vi "MiniCTA.vi"() -> ()   [LabVIEW 2020]
uses:
  controls/DIPSingleRadioButton.ctl
  controls/DIPBankRadioButton.ctl
  <vilib>/Utility/NIReport.llb/NI_ReportGenerationCore.lvlib
  <vilib>/printing/EasyPrintingControls.llb/report_type.ctl
  <vilib>/printing/EasyPrintingControls.llb/orientation.ctl
  <vilib>/printing/EasyPrintingControls.llb/panel_scaling_for_page.ctl
  <vilib>/printing/EasyPrintingControls.llb/margin_values.ctl
  <vilib>/printing/EasyPrintingControls.llb/measurement_system.ctl
  <vilib>/printing/EasyPrintingControls.llb/margins.ctl
  <vilib>/printing/EasyPrintingControls.llb/printing_method.ctl
  <vilib>/printing/EasyPrintingControls.llb/color_or_monochrome.ctl
  <vilib>/printing/EasyPrintingControls.llb/printer_options.ctl
  <vilib>/printing/EasyPrintingControls.llb/page_headers.ctl
  <vilib>/printing/EasyPrintingControls.llb/page_header_content_options.ctl
  <vilib>/printing/EasyPrintingControls.llb/page_header_options.ctl
  <vilib>/printing/EasyPrintingControls.llb/layout_options.ctl
  <vilib>/printing/EasyPrintingControls.llb/list_which_controls.ctl
  <vilib>/printing/EasyPrintingControls.llb/custom_contents_options.ctl
  <vilib>/printing/EasyPrinting.llb/Easy Print VI Panel or Documentation (path).vi
panel:
  in  "Tab Control":T1(tab)
  in  "Cable Length (m)":dbl=4.0 min=4.0 max=20.0 step=1.0
  out "SW1":T2
  out "SW2":T2
  out "SW3":T2
  out "ShortOK":bool
  out "ProbeOK":bool
  in  "Shorted Resistance":dbl min=0.0 max=2.0 step=0.1 format="%.2g"
  in  "Total Resistance":dbl min=0.0 max=100.0 step=0.1 format="%.2g"
  out "AllOK?":bool
  out "Cable Resistance":dbl format="%.2g"
  out "Filament\nHot Resistance":dbl format="%.2g"
  in  "Overheat":dbl=1.5
  out "Filament\nCold Resistance":dbl format="%.2g"
  out "TargetTotal\nHotResistance":dbl
  out "BridgeSetting":dbl
  out "Rbin":dbl
  out "SW1remainder":dbl
  out "n160":i32
  out "n20":i32
  out "SW2remainder":dbl
  out "n1.4":i32
  out "SW3remainder":dbl
  in  "alpha":dbl=0.0039
  out "Failed recipients":string[](array[string])
  in  "print?":bool
  in  "Recipients":string[](array[string])=["ttech@cppwind.com"]
  in  "Stop Button":bool
  in  "email?":bool
  # "1. Connect probe holder (sting or pigtail type) to 4-10m or 10-20m probe cable; SET DIP  SW1- 3 OR 4 appropriately\n2. Insert shorting probe.\n2. Use CEM DT-5302 (or alternative) Low Resistance Tester on 40 Ohm range to measure shorted holder and cable resistance, and enter displayed value on \"Basic\" tab.\n3. Remove shorting probe and insert hotfilm probe.\n4. Measure total resistance and enter displayed value on \"Basic\" tab, again using the 40 Ohm range setting. CAUTION! The 4 and 400 milliohm settings on the CEM DT-5302 drive large enough currents to damage the probe after a few seconds by heat dissipated through the probe.\n5. Set DIP switches as shown - a  dot indicating the switch should be pushed on that side.\n6. Connect the probe cable to the anemometer's \"Probe\" connection.\n7. Power up the bridge by plugging in PSU.\n\nOnly connect probe AFTER switches are set correctly. Power down before unplugging probe."
  # "="
  # "+"
  # "="
  # "X"
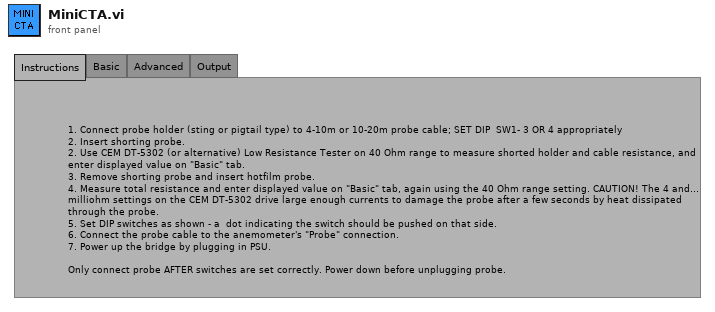
[diagram p1: front panel]
types:
  T1 = enum32{"Instructions", "Basic", "Advanced", "Output"}
  T2 = typedef "DIPBankRadioButton.ctl" = T3[]
  T3 = typedef "DIPSingleRadioButton.ctl" = enum32{"Radio Selection 1", "Radio Selection 2"}
  T4 = typedef "NI_ReportGenerationCore.lvlib/custom_contents_options.ctl" = cluster{"include VI connector and icon":bool, "include VI description":bool, "include front panel":bool, "surround front panel with border":bool, "list of controls options":cluster{"include list of controls":bool, "list which controls?":T5, "include control descriptions?":bool, "include control data types?":bool}, "block diagram options":cluster{"include block diagram":bool, "hidden frames":bool, "ordered (repeat from higher level if nested)":bool}, "include VI hierarchy":bool, "include list of subVIs":bool, "include VI history":bool, "include Express VI configuration information":bool}
  T5 = typedef "NI_ReportGenerationCore.lvlib/list_which_controls.ctl" = u16
  T6 = typedef "NI_ReportGenerationCore.lvlib/layout_options.ctl" = cluster{"orientation (unchanged)":T7, "panel scaling for page (unchanged)":T8, "margins":T9, "printer options":T12, "page header options":T15}
  T7 = typedef "NI_ReportGenerationCore.lvlib/orientation.ctl" = u16
  T8 = typedef "NI_ReportGenerationCore.lvlib/panel_scaling_for_page.ctl" = u16
  T9 = typedef "NI_ReportGenerationCore.lvlib/margins.ctl" = cluster{"override VI margins (false)":bool, "margins (1.00)":T10, "measurement system (default)":T11}
  T10 = typedef "NI_ReportGenerationCore.lvlib/margin_values.ctl" = cluster{"top":dbl, "left":dbl, "right":dbl, "bottom":dbl}
  T11 = typedef "NI_ReportGenerationCore.lvlib/measurement_system.ctl" = u16
  T12 = typedef "NI_ReportGenerationCore.lvlib/printer_options.ctl" = cluster{"destination printer name (current)":string, "printing method (unchanged)":T13, "color or monochrome (unchanged)":T14}
  T13 = typedef "NI_ReportGenerationCore.lvlib/printing_method.ctl" = u16
  T14 = typedef "NI_ReportGenerationCore.lvlib/color_or_monochrome.ctl" = u16
  T15 = typedef "NI_ReportGenerationCore.lvlib/page_header_options.ctl" = cluster{"page headers (unchanged)":T16, "page header content options":T17}
  T16 = typedef "NI_ReportGenerationCore.lvlib/page_headers.ctl" = u16
  T17 = typedef "NI_ReportGenerationCore.lvlib/page_header_content_options.ctl" = cluster{"Include VI Name":bool, "Include VI Path":bool, "Include Last Modification Date":bool, "Include Date Printed":bool, "Include Page Number":bool, "Include VI Icon":bool}
  T18 = typedef "NI_ReportGenerationCore.lvlib/report_type.ctl" = u16
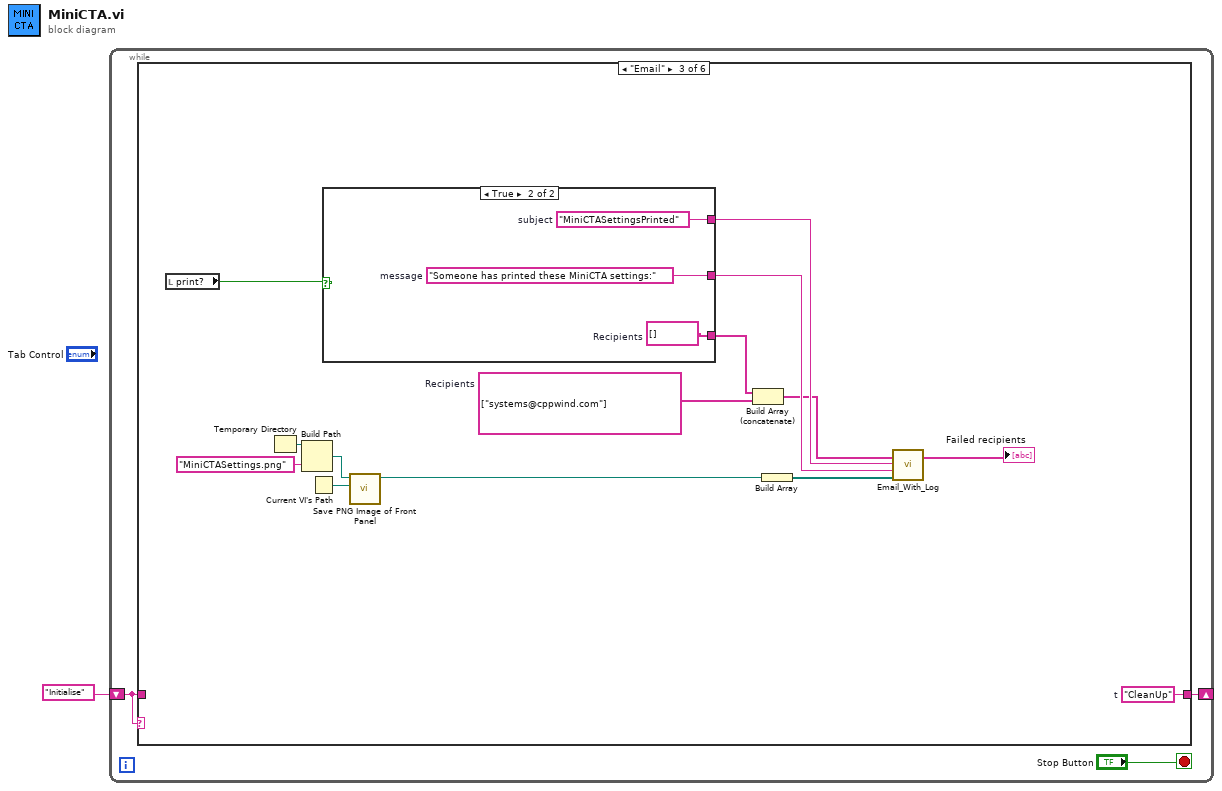
[diagram p0: block diagram]
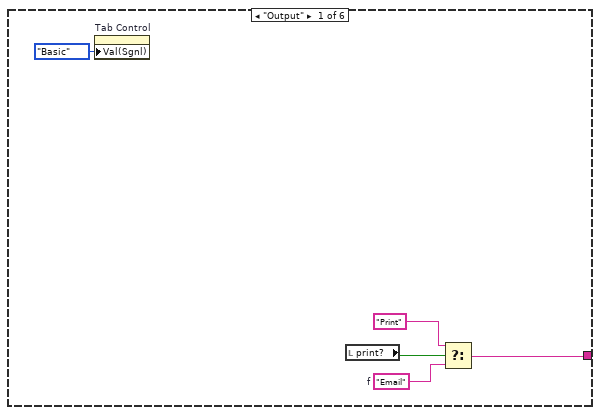
[diagram p2: hidden frame]
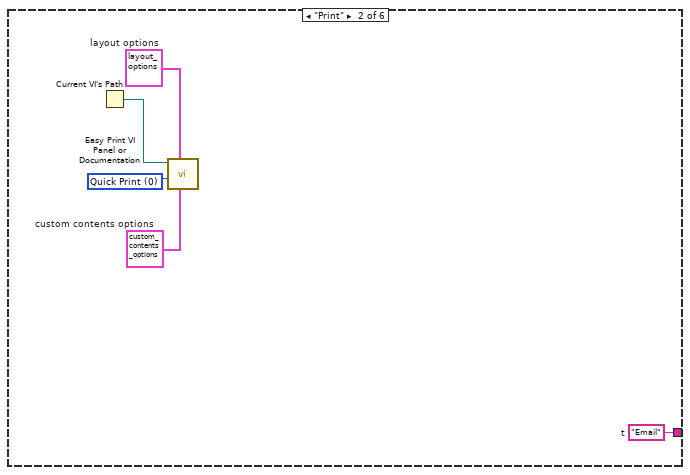
[diagram p3: hidden frame]
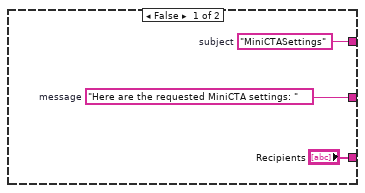
[diagram p4: hidden frame]
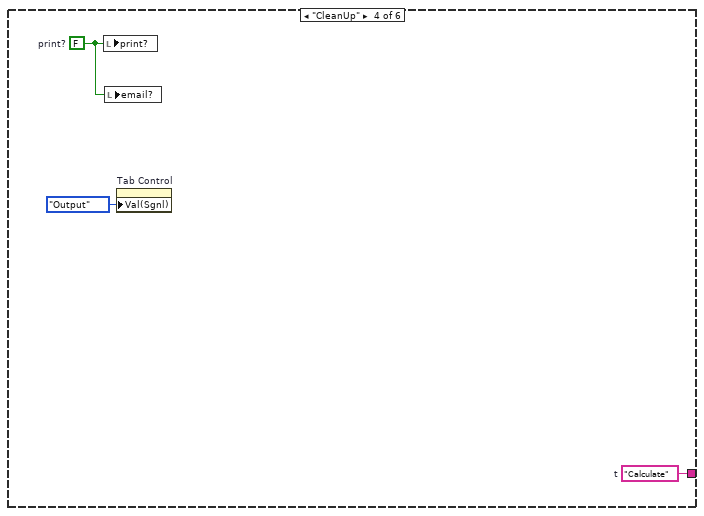
[diagram p5: hidden frame]
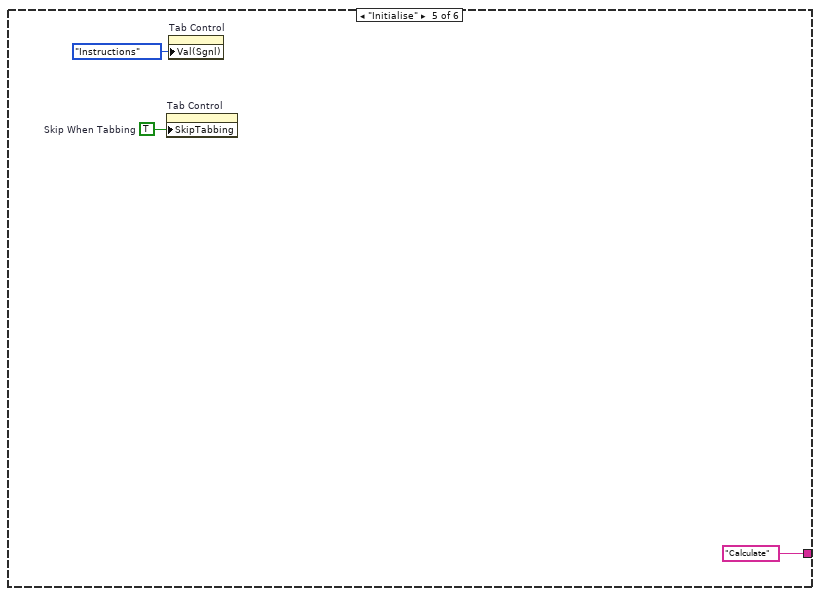
[diagram p6: hidden frame]
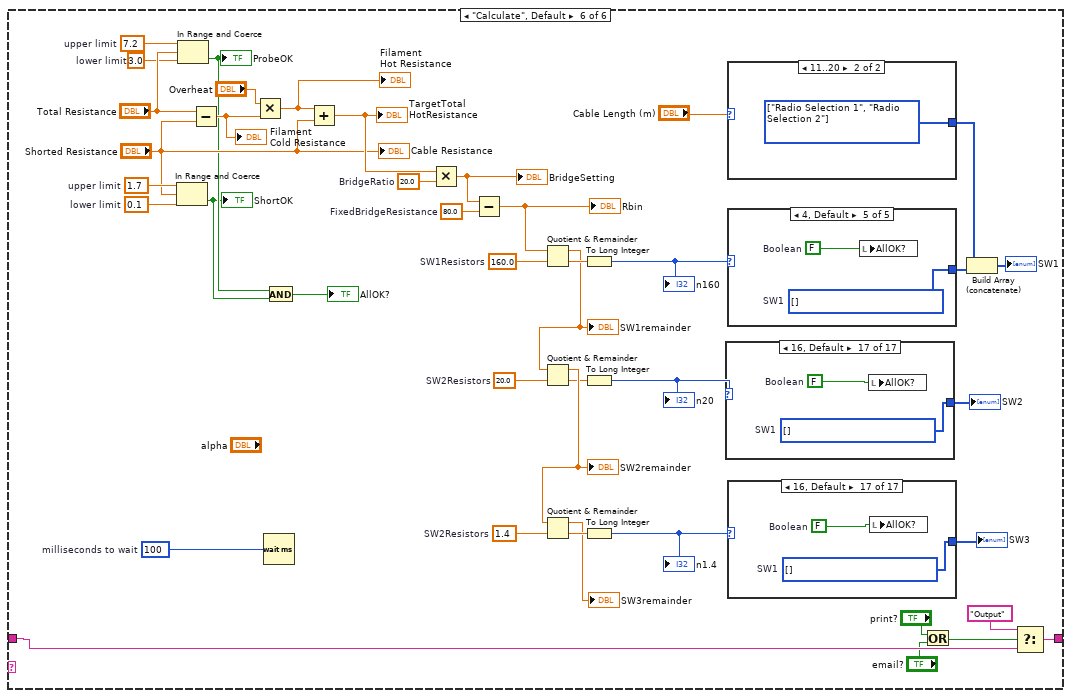
[diagram p7: hidden frame]
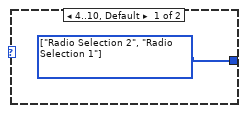
[diagram p8: hidden frame]
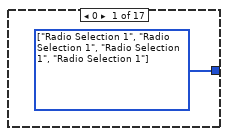
[diagram p9: hidden frame]
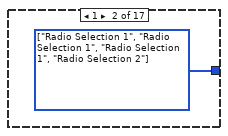
[diagram p10: hidden frame]
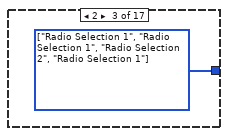
[diagram p11: hidden frame]
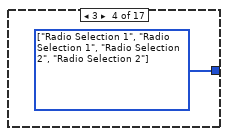
[diagram p12: hidden frame]
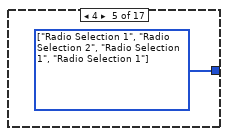
[diagram p13: hidden frame]
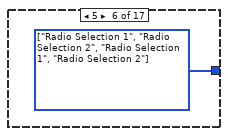
[diagram p14: hidden frame]
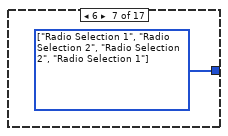
[diagram p15: hidden frame]
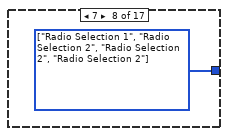
[diagram p16: hidden frame]
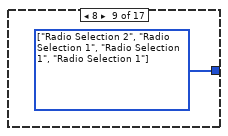
[diagram p17: hidden frame]
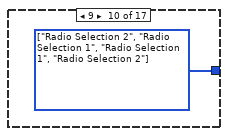
[diagram p18: hidden frame]
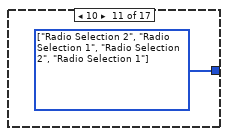
[diagram p19: hidden frame]
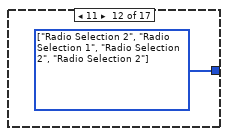
[diagram p20: hidden frame]
diagram:
  n1 = while {
    shift-right: [w2] -> _
    shift-left: "Initialise" -> [w3]
    stop <- "Stop Button" stop-if-true
    n2 = case shown="\"Email\"" w3 {
      tunnel: w3 -> [_ _ _ _ _ w50]
      tunnel: [w8 w13 w28 w36 "Calculate" w51] -> w2
      frame "Output" {
        w5 = "Email"  # f
        n3 = property on="Tab Control" class="TabCtl (strict)"("Val(Sgnl)"=T1."Basic" ("Value (Signaling)")) -> ()  [unwired: 2 in, 2 out]
        n4 = local read "print?"() -> (w7:bool)
        n5 = Select(t="Print", s=w7, f=w5) -> (s? t:f=w8:string)
      }
      frame "Print" {
        w10 = T4 {"include VI connector and icon"=FALSE, "include VI description"=FALSE, "include front panel"=FALSE, "surround front panel with border"=FALSE, "list of controls options"={"include list of controls"=FALSE, "list which controls?"=0, "include control descriptions?"=FALSE, "include control data types?"=FALSE}, "block diagram options"={"include block diagram"=FALSE, "hidden frames"=FALSE, "ordered (repeat from higher level if nested)"=FALSE}, "include VI hierarchy"=FALSE, "include list of subVIs"=FALSE, "include VI history"=FALSE, "include Express VI configuration information"=FALSE}  # custom contents options
        w11 = T6 {"orientation (unchanged)"=0, "panel scaling for page (unchanged)"=0, "margins"={"override VI margins (false)"=FALSE, "margins (1.00)"={"top"=1.0, "left"=1.0, "right"=1.0, "bottom"=1.0}, "measurement system (default)"=0}, "printer options"={"destination printer name (current)"="", "printing method (unchanged)"=0, "color or monochrome (unchanged)"=0}, "page header options"={"page headers (unchanged)"=1, "page header content options"={"Include VI Name"=FALSE, "Include VI Path"=FALSE, "Include Last Modification Date"=FALSE, "Include Date Printed"=TRUE, "Include Page Number"=FALSE, "Include VI Icon"=FALSE}}}  # layout options
        w12 = T18 0 items=["Quick Print", "Standard Report", "HTML", "Word", "Excel"] ("report type (Quick Print)")
        w13 = "Email"  # t
        n6 = Current VI's Path() -> (path=w14:path)
        n7 = call-poly <vilib>:"Easy Print VI Panel or Documentation.vi"("custom contents options"=w10, "layout options"=w11, "report type (Quick Print)"=w12, "VI path"=w14) -> ()  [unwired: 6 in, 2 out]
      }
      frame "Email" {
        w24 = string[] ["systems@cppwind.com"]  # Recipients
        w28 = "CleanUp"  # t
        n8 = local read "print?"() -> (w21:bool)
        n9 = Temporary Directory() -> (w27:path)
        n10 = Build Path(base path=w27, name or relative path="MiniCTASettings.png") -> (appended path=w26:path)
        n11 = Current VI's Path() -> (path=w22:path)
        n12 = case shown="True" w21 {
          tunnel: ["Recipients" w34] -> w23
          tunnel: [w30 w33] -> w18
          tunnel: [w29 w32] -> w19
          frame False {
            w29 = "Here are the requested MiniCTA settings: "  # message
            w30 = "MiniCTASettings"  # subject
          }
          frame True {
            w32 = "Someone has printed these MiniCTA settings:"  # message
            w33 = "MiniCTASettingsPrinted"  # subject
            w34 = string[] []  # Recipients
          }
        }
        n13 = call "Save PNG Image of Front Panel.vi"("VI Path"=w22, "File Path In"=w26) -> ("File Path Out"=w15:path)  [unwired: 8 in, 1 out]
        n14 = Build Array (concatenate)(w23, w24) -> (w17:string[])
        n15 = Build Array(w15) -> (w20:path[])
        n16 = call "Email_With_Log.vi"("recipients"=w17, "subject ([No Subject])"=w18, "message"=w19, "attachments"=w20) -> ("invalid recipients"=→"Failed recipients":string[])  [unwired: 1 in, 1 out]
      }
      frame "CleanUp" {
        w36 = "Calculate"  # t
        w37 = FALSE  # print?
        n17 = local write "print?"(w37) -> ()
        n18 = local write "email?"(w37) -> ()
        n19 = property on="Tab Control" class="TabCtl (strict)"("Val(Sgnl)"=T1."Output" ("Value (Signaling)")) -> ()  [unwired: 2 in, 2 out]
      }
      frame "Initialise" {
        w38 = TRUE  # Skip When Tabbing
        n20 = property on="Tab Control" class="TabCtl (strict)"("SkipTabbing"=w38) -> ()  [unwired: 2 in, 2 out]
        n21 = property on="Tab Control" class="TabCtl (strict)"("Val(Sgnl)"=T1."Instructions" ("Value (Signaling)")) -> ()  [unwired: 2 in, 2 out]
      }
      frame "Calculate", Default {
        w55 = 7.2  # upper limit
        w56 = 3.0  # lower limit
        w58 = 0.1  # lower limit
        w59 = 1.7  # upper limit
        w60 = u32 100  # milliseconds to wait
        w69 = 1.4  # SW2Resistors
        w72 = 20.0  # SW2Resistors
        w75 = 160.0  # SW1Resistors
        w77 = 80.0  # FixedBridgeResistance
        w79 = 20.0  # BridgeRatio
        n22 = In Range and Coerce(upper limit=w59, x="Shorted Resistance", lower limit=w58) -> (In Range?=w42:bool)  [unwired: 1 out]
        "ShortOK" <- w42
        n23 = In Range and Coerce(upper limit=w55, x="Total Resistance", lower limit=w56) -> (In Range?=w43:bool)  [unwired: 1 out]
        "ProbeOK" <- w43
        n24 = Subtract(x="Total Resistance", y="Shorted Resistance") -> (x-y=w82:dbl)
        "Filament\nCold Resistance" <- w82
        n25 = Multiply(x="Overheat", y=w82) -> (x*y=w45:dbl)
        "Filament\nHot Resistance" <- w45
        n26 = Wait (ms)(milliseconds to wait=w60) -> ()  [unwired: 1 out]
        n27 = And(x=w43, y=w42) -> (x .and. y?=→"AllOK?":bool)
        n28 = Add(x=w45, y="Shorted Resistance") -> (x+y=w80:dbl)
        "TargetTotal\nHotResistance" <- w80
        n29 = Multiply(x=w80, y=w79) -> (x*y=w78:dbl)
        "BridgeSetting" <- w78
        n30 = Subtract(x=w78, y=w77) -> (x-y=w76:dbl)
        "Rbin" <- w76
        n31 = Quotient & Remainder(x=w76, y=w75) -> (x-y*floor(x/y)=w71:dbl, floor(x/y)=w74:dbl)
        "SW1remainder" <- w71
        n32 = Quotient & Remainder(x=w71, y=w72) -> (x-y*floor(x/y)=w68:dbl, floor(x/y)=w65:dbl)
        "SW2remainder" <- w68
        n33 = Quotient & Remainder(x=w68, y=w69) -> (x-y*floor(x/y)=→"SW3remainder":dbl, floor(x/y)=w63:dbl)
        n34 = To Long Integer(number=w74) -> (32bit integer=w66:i32)
        "n160" <- w66
        n35 = To Long Integer(number=w65) -> (32bit integer=w64:i32)
        "n20" <- w64
        n36 = To Long Integer(number=w63) -> (32bit integer=w62:i32)
        "n1.4" <- w62
        n37 = case shown="16, Default" w64 {
          tunnel: [w103 w104 w105 w106 w107 w108 w109 w110 w111 w112 w113 w114 w115 w116 w117 w118 w120] -> w70
          frame 0 {
            w103 = T2 [enum."Radio Selection 1", enum."Radio Selection 1", enum."Radio Selection 1", enum."Radio Selection 1"] items=["Radio Selection 1", "Radio Selection 2"] ("SW1")
          }
          frame 1 {
            w104 = T2 [enum."Radio Selection 1", enum."Radio Selection 1", enum."Radio Selection 1", enum."Radio Selection 2"] items=["Radio Selection 1", "Radio Selection 2"] ("SW1")
          }
          frame 2 {
            w105 = T2 [enum."Radio Selection 1", enum."Radio Selection 1", enum."Radio Selection 2", enum."Radio Selection 1"] items=["Radio Selection 1", "Radio Selection 2"] ("SW1")
          }
          frame 3 {
            w106 = T2 [enum."Radio Selection 1", enum."Radio Selection 1", enum."Radio Selection 2", enum."Radio Selection 2"] items=["Radio Selection 1", "Radio Selection 2"] ("SW1")
          }
          frame 4 {
            w107 = T2 [enum."Radio Selection 1", enum."Radio Selection 2", enum."Radio Selection 1", enum."Radio Selection 1"] items=["Radio Selection 1", "Radio Selection 2"] ("SW1")
          }
          frame 5 {
            w108 = T2 [enum."Radio Selection 1", enum."Radio Selection 2", enum."Radio Selection 1", enum."Radio Selection 2"] items=["Radio Selection 1", "Radio Selection 2"] ("SW1")
          }
          frame 6 {
            w109 = T2 [enum."Radio Selection 1", enum."Radio Selection 2", enum."Radio Selection 2", enum."Radio Selection 1"] items=["Radio Selection 1", "Radio Selection 2"] ("SW1")
          }
          frame 7 {
            w110 = T2 [enum."Radio Selection 1", enum."Radio Selection 2", enum."Radio Selection 2", enum."Radio Selection 2"] items=["Radio Selection 1", "Radio Selection 2"] ("SW1")
          }
          frame 8 {
            w111 = T2 [enum."Radio Selection 2", enum."Radio Selection 1", enum."Radio Selection 1", enum."Radio Selection 1"] items=["Radio Selection 1", "Radio Selection 2"] ("SW1")
          }
          frame 9 {
            w112 = T2 [enum."Radio Selection 2", enum."Radio Selection 1", enum."Radio Selection 1", enum."Radio Selection 2"] items=["Radio Selection 1", "Radio Selection 2"] ("SW1")
          }
          frame 10 {
            w113 = T2 [enum."Radio Selection 2", enum."Radio Selection 1", enum."Radio Selection 2", enum."Radio Selection 1"] items=["Radio Selection 1", "Radio Selection 2"] ("SW1")
          }
          frame 11 {
            w114 = T2 [enum."Radio Selection 2", enum."Radio Selection 1", enum."Radio Selection 2", enum."Radio Selection 2"] items=["Radio Selection 1", "Radio Selection 2"] ("SW1")
          }
          frame 12 {
            w115 = T2 [enum."Radio Selection 2", enum."Radio Selection 2", enum."Radio Selection 1", enum."Radio Selection 1"] items=["Radio Selection 1", "Radio Selection 2"] ("SW1")
          }
          frame 13 {
            w116 = T2 [enum."Radio Selection 2", enum."Radio Selection 2", enum."Radio Selection 1", enum."Radio Selection 2"] items=["Radio Selection 1", "Radio Selection 2"] ("SW1")
          }
          frame 14 {
            w117 = T2 [enum."Radio Selection 2", enum."Radio Selection 2", enum."Radio Selection 2", enum."Radio Selection 1"] items=["Radio Selection 1", "Radio Selection 2"] ("SW1")
          }
          frame 15 {
            w118 = T2 [enum."Radio Selection 2", enum."Radio Selection 2", enum."Radio Selection 2", enum."Radio Selection 2"] items=["Radio Selection 1", "Radio Selection 2"] ("SW1")
          }
          frame 16, Default {
            w119 = FALSE  # Boolean
            w120 = T2 [] items=["Radio Selection 1", "Radio Selection 2"]  # SW1
            n38 = local write "AllOK?"(w119) -> ()
          }
        }
        "SW2" <- w70
        n39 = case shown="11..20" "Cable Length (m)" {
          tunnel: [w83 w84] -> w52
          frame 4..10, Default {
            w83 = T2 [enum."Radio Selection 2", enum."Radio Selection 1"] items=["Radio Selection 1", "Radio Selection 2"] ("SW1")
          }
          frame 11..20 {
            w84 = T2 [enum."Radio Selection 1", enum."Radio Selection 2"] items=["Radio Selection 1", "Radio Selection 2"] ("SW1")
          }
        }
        n40 = case shown="4, Default" w66 {
          tunnel: [w121 w122 w123 w124 w126] -> w73
          frame 0 {
            w121 = T2 [enum."Radio Selection 1", enum."Radio Selection 1"] items=["Radio Selection 1", "Radio Selection 2"] ("SW1")
          }
          frame 1 {
            w122 = T2 [enum."Radio Selection 1", enum."Radio Selection 2"] items=["Radio Selection 1", "Radio Selection 2"] ("SW1")
          }
          frame 2 {
            w123 = T2 [enum."Radio Selection 2", enum."Radio Selection 2"] items=["Radio Selection 1", "Radio Selection 2"] ("SW1")
          }
          frame 3 {
            w124 = T2 [enum."Radio Selection 1", enum."Radio Selection 1"] items=["Radio Selection 1", "Radio Selection 2"] ("SW1")
          }
          frame 4, Default {
            w125 = FALSE  # Boolean
            w126 = T2 [] items=["Radio Selection 1", "Radio Selection 2"]  # SW1
            n41 = local write "AllOK?"(w125) -> ()
          }
        }
        n42 = case shown="16, Default" w62 {
          tunnel: [w85 w86 w87 w88 w89 w90 w91 w92 w93 w94 w95 w96 w97 w98 w99 w100 w102] -> w67
          frame 0 {
            w85 = T2 [enum."Radio Selection 1", enum."Radio Selection 1", enum."Radio Selection 1", enum."Radio Selection 1"] items=["Radio Selection 1", "Radio Selection 2"] ("SW1")
          }
          frame 1 {
            w86 = T2 [enum."Radio Selection 1", enum."Radio Selection 1", enum."Radio Selection 1", enum."Radio Selection 2"] items=["Radio Selection 1", "Radio Selection 2"] ("SW1")
          }
          frame 2 {
            w87 = T2 [enum."Radio Selection 1", enum."Radio Selection 1", enum."Radio Selection 2", enum."Radio Selection 1"] items=["Radio Selection 1", "Radio Selection 2"] ("SW1")
          }
          frame 3 {
            w88 = T2 [enum."Radio Selection 1", enum."Radio Selection 1", enum."Radio Selection 2", enum."Radio Selection 2"] items=["Radio Selection 1", "Radio Selection 2"] ("SW1")
          }
          frame 4 {
            w89 = T2 [enum."Radio Selection 1", enum."Radio Selection 2", enum."Radio Selection 1", enum."Radio Selection 1"] items=["Radio Selection 1", "Radio Selection 2"] ("SW1")
          }
          frame 5 {
            w90 = T2 [enum."Radio Selection 1", enum."Radio Selection 2", enum."Radio Selection 1", enum."Radio Selection 2"] items=["Radio Selection 1", "Radio Selection 2"] ("SW1")
          }
          frame 6 {
            w91 = T2 [enum."Radio Selection 1", enum."Radio Selection 2", enum."Radio Selection 2", enum."Radio Selection 1"] items=["Radio Selection 1", "Radio Selection 2"] ("SW1")
          }
          frame 7 {
            w92 = T2 [enum."Radio Selection 1", enum."Radio Selection 2", enum."Radio Selection 2", enum."Radio Selection 2"] items=["Radio Selection 1", "Radio Selection 2"] ("SW1")
          }
          frame 8 {
            w93 = T2 [enum."Radio Selection 2", enum."Radio Selection 1", enum."Radio Selection 1", enum."Radio Selection 1"] items=["Radio Selection 1", "Radio Selection 2"] ("SW1")
          }
          frame 9 {
            w94 = T2 [enum."Radio Selection 2", enum."Radio Selection 1", enum."Radio Selection 1", enum."Radio Selection 2"] items=["Radio Selection 1", "Radio Selection 2"] ("SW1")
          }
          frame 10 {
            w95 = T2 [enum."Radio Selection 2", enum."Radio Selection 1", enum."Radio Selection 2", enum."Radio Selection 1"] items=["Radio Selection 1", "Radio Selection 2"] ("SW1")
          }
          frame 11 {
            w96 = T2 [enum."Radio Selection 2", enum."Radio Selection 1", enum."Radio Selection 2", enum."Radio Selection 2"] items=["Radio Selection 1", "Radio Selection 2"] ("SW1")
          }
          frame 12 {
            w97 = T2 [enum."Radio Selection 2", enum."Radio Selection 2", enum."Radio Selection 1", enum."Radio Selection 1"] items=["Radio Selection 1", "Radio Selection 2"] ("SW1")
          }
          frame 13 {
            w98 = T2 [enum."Radio Selection 2", enum."Radio Selection 2", enum."Radio Selection 1", enum."Radio Selection 2"] items=["Radio Selection 1", "Radio Selection 2"] ("SW1")
          }
          frame 14 {
            w99 = T2 [enum."Radio Selection 2", enum."Radio Selection 2", enum."Radio Selection 2", enum."Radio Selection 1"] items=["Radio Selection 1", "Radio Selection 2"] ("SW1")
          }
          frame 15 {
            w100 = T2 [enum."Radio Selection 2", enum."Radio Selection 2", enum."Radio Selection 2", enum."Radio Selection 2"] items=["Radio Selection 1", "Radio Selection 2"] ("SW1")
          }
          frame 16, Default {
            w101 = FALSE  # Boolean
            w102 = T2 [] items=["Radio Selection 1", "Radio Selection 2"]  # SW1
            n43 = local write "AllOK?"(w101) -> ()
          }
        }
        "SW3" <- w67
        n44 = Or(x="print?", y="email?") -> (x .or. y?=w47:bool)
        n45 = Build Array (concatenate)(w52, w73) -> (→"SW1":T2)
        n46 = Select(t="Output", s=w47, f=w50) -> (s? t:f=w51:string)
        "Cable Resistance" <- "Shorted Resistance"
      }
    }
  }
